vi "LIA.SR810.SetResource.vi"(8 "error in (no error)":errorcluster, 10 "Resource":T1, 11 "LIA.SR810 in":refnum<class "LIA.SR810.lvclass">) -> (0 "error out":errorcluster, 3 "LIA.SR810 out":refnum<class "LIA.SR810.lvclass">)   [LabVIEW 2017, in "LIA.SR810.lvclass"]
uses:
  LIA.SR810.lvclass
  LIA.SR810.lvclass/LIA.SR810.ctl
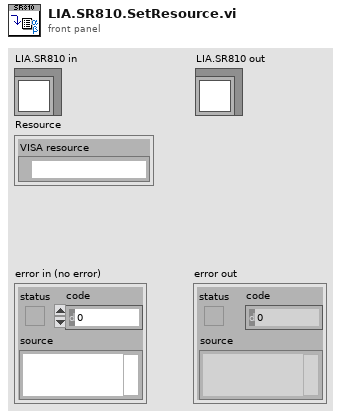
[diagram p1: front panel]
types:
  T1 = cluster{"VISA resource":refnum<visa-resource-name>}
  T2 = typedef "LIA.SR810.lvclass/PrivateData--Ref.ctl" = refnum<data-value>
  T3 = typedef "LIA.SR810.lvclass/PrivateData--Cluster.ctl" = cluster{"Resource":cluster{"VISA resource":refnum<visa-resource-name>}}
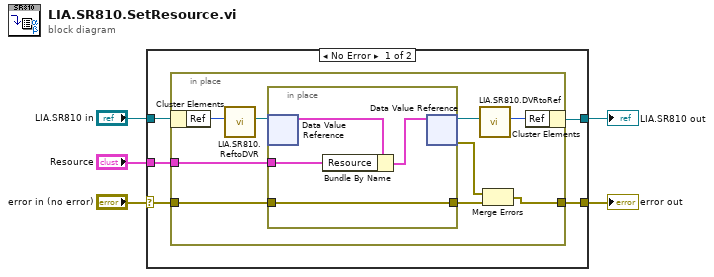
[diagram p0: block diagram]
diagram:
  n1 = case shown="No Error" "error in (no error)" {
    selector: "error in (no error)" -> [w7 w25]
    tunnel: [w6 w25] -> w4
    tunnel: [w8 w24] -> w2
    tunnel: "LIA.SR810 in" -> [w10 w24]
    tunnel: "Resource" -> [w9 _]
    frame No Error {
      n2 = in-place {
        in-place-border: w9 -> [w15]
        in-place-border: w7 -> [w14]
        in-place-border: [w11] -> w6
        n3 = in-place-cluster #1(w10) -> ("Ref"=w19:u32)
        n4 = call "LIA.SR810.ReftoDVR.vi"("Ref"=w19) -> ("Ref"=w16:T2)  [unwired: 10 in]
        n5 = in-place {
          in-place-border: w15 -> [w22]
          in-place-border: w14 -> [w20]
          in-place-border: [w20] -> w12
          n6 = in-place-dvr #2(w16) -> (w23:T3)  [unwired: 1 out]
          n7 = Bundle By Name(cluster=w23, "Resource"=w22) -> (w21:T3)
          n8 = in-place-dvr #2(w21) -> (w17:T2, w13:errorcluster)
        }
        n9 = call "LIA.SR810.DVRtoRef.vi"("Ref"=w17) -> ("Ref"=w18:u32)  [unwired: 10 in]
        n10 = Merge Errors(w13, w12) -> (w11:errorcluster)
        n11 = in-place-cluster #1("Ref"=w18) -> (w8:refnum<class "LIA.SR810.lvclass">)
      }
    }
    frame Error {
    }
  }
  "error out" <- w4
  "LIA.SR810 out" <- w2
